vi "step.vi"(8 "error in (no error)":errorcluster, 11 "object in":refnum<class "SQLiteConnection.lvclass">) -> (0 "error out":errorcluster, 2 "row?":bool, 3 "object out":refnum<class "SQLiteConnection.lvclass">)   [LabVIEW 2019, in "SQLiteConnection.lvclass"]
uses:
  SQLiteConnection.lvclass
  SQLiteConnection.lvclass/SQLiteConnection.ctl
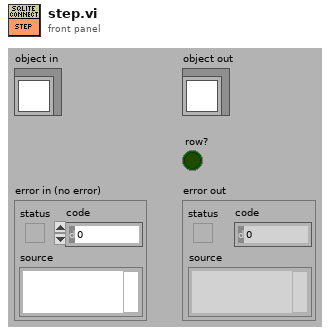
[diagram p1: front panel]
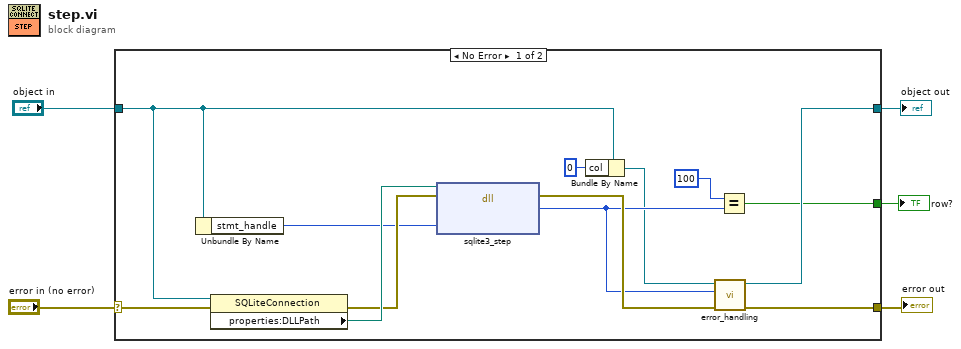
[diagram p0: block diagram]
diagram:
  n1 = case shown="No Error" "error in (no error)" {
    selector: "error in (no error)" -> [w16 w20]
    tunnel: [w18 w20] -> w4
    tunnel: [w17 w19] -> w2
    tunnel: "object in" -> [w8 w19]
    tunnel: [w10 _] -> w1
    frame No Error {
      n2 = Unbundle By Name(w8) -> ("stmt_handle"=w12:u64)
      n3 = property class="SQLiteConnection"(reference=w8, error in=w16) -> (error out=w14:errorcluster, "properties:DLLPath"=w15:path)  [unwired: 1 out]
      n4 = dll-call lib="D:/Users/mcarl/Documents/LabVIEW Projects/OW-PIKO/OW-PIKO Software/sqlite3.dll" fn="sqlite3_step"(path in=w15, error in=w14, "stmt_pointer"=w12) -> (error out=w13:errorcluster, "return type"=w11:i32)  [unwired: 2 in, 1 out]
      n5 = Bundle By Name(cluster=w8, "col"=0) -> (w7:refnum<class "SQLiteConnection.lvclass">)
      n6 = call "error_handling.vi"("error in (no error)"=w13, "error handle"=w11, "object in"=w7) -> ("error out"=w18:errorcluster, "object out"=w17:refnum<class "SQLiteConnection.lvclass">)  [unwired: 7 in]
      n7 = Equal?(x=100, y=w11) -> (x = y?=w10:bool)
    }
    frame Error {
    }
  }
  "error out" <- w4
  "object out" <- w2
  "row?" <- w1
